vi "CSGaussmeter.initialize.vi"(0 "i ref in":refnum<vi>, 11 "error in":errorcluster) -> (4 "i ref out":refnum<vi>, 15 "error out":errorcluster)   [LabVIEW 2014, in "CSGaussmeter.lvlib"]
doc: "Durch das VI init wird das Gerät neu initalisiert\n\nThe VI initializes the device"
uses:
  CSGaussmeter.lvlib
  CS_Core/CSObj/CSObj.lvlib
  CSlibraries/UtilityLib/UtilityLib.lvlib
  instr.lib/FH_55/FH 55.lvlib
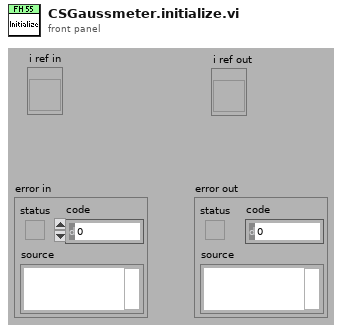
[diagram p1: front panel]
types:
  T1 = typedef "CSGaussmeter.lvlib/CSGaussmeter.i attribute.ctl" = cluster{"Name":string, "VISA Resource Name":refnum<visa-resource-name>, "actValues":cluster{" Limit":bool, "Unit ":T2, "Temp_Unit":T3, "Max":T4, " Filter":bool, " Peak":bool, " Auto_Range":bool, "Range":T5, " Rel":bool, " CTemp":bool, " CField":bool, "AC_DC ":bool, "Set_lower":cluster{"Numeric":dbl, "Cancel Button":bool, "Unit":T6}, "Set_upper":cluster{"Numeric":dbl, "Cancel Button":bool, "Unit":T6}, "Set_Rel":cluster{"Numeric":dbl, "Cancel Button":bool, "Unit":T6}, "Zero":bool, " Local":bool, "Reset":bool, " Init":bool}, "FH 55 Gauss-/Teslameter":T7, "MAX_Value":T8, "MIN_Value":T8, "Rel_Value":T8, "Array ":string[], "LIMU":dbl, " LIML":dbl, "Messwerte 2":string, "Messwerte ":cluster{"Numeric":i32, "OK Button":bool}, "serviceID":cluster{"Current ID":i32, "Unit ID":i32, "Temp ID":i32, "Name ID \n":i32, "Visa ID ":i32}, "setValues ":cluster{" Limit":bool, "Unit ":T2, "Temp_Unit":T3, "Max":T4, " Filter":bool, " Peak":bool, " Auto_Range":bool, "Range":T5, " Rel":bool, " CTemp":bool, " CField":bool, "AC_DC ":bool, "Set_lower":cluster{"Numeric":dbl, "Cancel Button":bool, "Unit":T6}, "Set_upper":cluster{"Numeric":dbl, "Cancel Button":bool, "Unit":T6}, "Set_Rel":cluster{"Numeric":dbl, "Cancel Button":bool, "Unit":T6}, "Zero":bool, " Local":bool, "Reset":bool, " Init":bool}}
  T2 = typedef "FH 55.lvlib/Unit.ctl" = enum16{"T", "G", "A/m"}
  T3 = typedef "FH 55.lvlib/Temp_Unit.ctl" = enum16{"Temp off", "Celsius", "Fahrenheit"}
  T4 = typedef "FH 55.lvlib/Max.ctl" = enum16{"MAX off", "Show MAX", "MAX/MIN"}
  T5 = typedef "FH 55.lvlib/Range.ctl" = enum16{"1", "2", "3", "4", "5", "6", "7"}
  T6 = typedef "FH 55.lvlib/Unit2.ctl" = enum16{"mT", "G", "kA/m"}
  T7 = typedef "FH 55.lvlib/Display.ctl" = cluster{"current value":string, "Limit":string, "Remote":string, "function ":string, "Cluster":cluster{"AC/DC":string, "Auto":string, "Filter":string, "Range":string, "Rel":string, "Peak":string}}
  T8 = typedef "FH 55.lvlib/Value_String.ctl" = cluster{"Numeric":dbl, "String":string}
  T9 = cluster{"VISA Resource Name":refnum<visa-resource-name>}
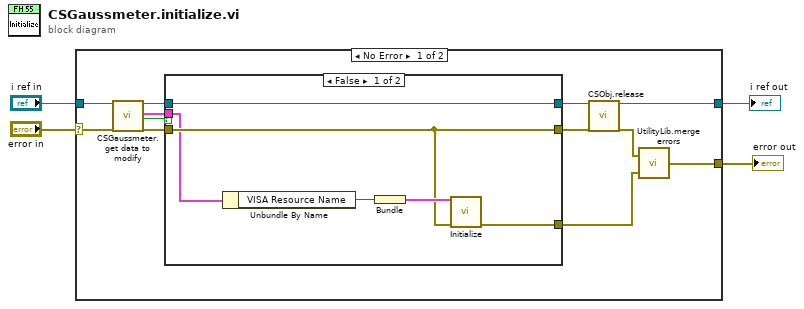
[diagram p0: block diagram]
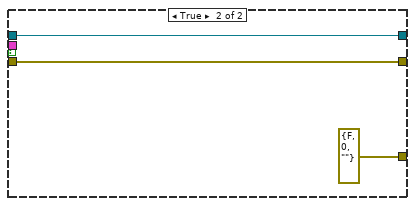
[diagram p2: hidden frame]
diagram:
  n1 = case shown="No Error" "error in" {
    selector: "error in" -> [w10 w26]
    tunnel: "i ref in" -> [w11 w27]
    tunnel: [w5 w27] -> w2
    tunnel: [w12 w26] -> w1
    frame No Error {
      n2 = call "CSGaussmeter.get data to modify.vi"("i ref in"=w11, "error in (no error)"=w10) -> ("i ref out"=w6:refnum<vi>, "i attribute"=w7:T1, "timed out"=w8:bool, "error out"=w9:errorcluster)  [unwired: 14 in]
      n3 = case shown="False" w8 {
        tunnel: w6 -> [w21 w23]
        tunnel: w9 -> [w19 w25]
        tunnel: w7 -> [w17 _]
        tunnel: [w19 w25] -> w15
        tunnel: [w18 errorcluster {"status"=FALSE, "code"=0, "source"=""} ("error out")] -> w16
        tunnel: [w21 w23] -> w13
        frame False {
          n4 = Unbundle By Name(w17) -> ("VISA Resource Name"=w22:refnum<visa-resource-name>)
          n5 = Bundle("VISA Resource Name"=w22) -> (w20:T9)  [unwired: 1 in]
          n6 = call "Initialize.vi"("VisaCluster"=w20, "error in (no error)"=w19) -> ("error out"=w18:errorcluster)  [unwired: 12 in, 1 out]
        }
        frame True {
        }
      }
      n7 = call "CSObj.release.vi"("i ref in"=w13, "error in (no error)"=w15) -> ("i ref out"=w5:refnum<vi>, "error out"=w14:errorcluster)  [unwired: 16 in]
      n8 = call "UtilityLib.merge errors.vi"("error2 (no error)"=w16, "error1 (no error)"=w14) -> ("error out"=w12:errorcluster)
    }
    frame Error {
    }
  }
  "i ref out" <- w2
  "error out" <- w1
